vi "Couple Head Impulse Traces.vi"(0 "Data Input":T5 {"Data Channels" format="%.2f"}, 1 "Impulse Positions":T1(array[cluster]) {"Amplitude offset" format="%.2f"}, 2 "Trace Select":i32 min=0 max=1000, 3 "Impulse Direction +ve?":bool, 4 "Capture Saccade":bool, 5 "Impulse Plane":T4(ring), 6 "Mean and STD":bool, 7 "Plot Selection 2":T3 {"Gain" format="%.1f"; "Offset" format="%.1f"}, 8 "Export":bool, 9 "desacc":T2={"Threshold 1 [Acc]"=0.0, "Threshold 2 [% of TH1]"=0, "tolerance"=2, "Search WD "=0.05757575757575758, " always use TH2"=TRUE, "Range"=3.0303030303030303, "Max time"=50.0, "Min time"=1.0, "Velocity Threshold"=0} {"Velocity Threshold" scale=0.0..100.0; "Range" scale=0.0..5.0; "Search WD" scale=0.0..0.3; "tolerance" scale=0.0..10.0; "Threshold 2 [% of TH1]" scale=0.0..100.0; "Threshold 1 [Acc]" scale=1.0..20000.0}, 10 "Interpolate":bool, 13 "S-pline":bool, 15 "desacc.":bool=TRUE, 16 "man. desacc..":bool, 17 "Display Saccade":bool, 18 "balance parameter (s-pline Parameter)":dbl(slide)=0.9 min=0.8 max=1.0 step=0.0001 scale=0.8..1.0) -> (11 "Impulse Positions 2":T1(array[cluster]) {"Amplitude offset" format="%.2f"}, 12 "No Impulses":i32, 14 "Impulses":dbl[][](graph), 19 "Mean and STD":dbl[][](array[numeric]) format="%.2f")   [LabVIEW 2016, in "impulse functions.lvlib"]
uses:
  impulse functions.lvlib
  core/type-defs/TD_Impulse Parameter.ctl
  core/type-defs/TD_Impulse Planes.ctl
  <vilib>/Analysis/1siggen.llb/Ramp Pattern by Samples.vi
  stats/stats.lvlib
  <vilib>/Analysis/NI_AALPro.lvlib
  <vilib>/Analysis/NI_AALBase.lvlib
  core/core.lvlib
panel:
  out "Desaccaded 2":dbl[][](graph)
  # "Copyright Americo A. Migliaccio (c) 2002 All Rights Reserved by Author"
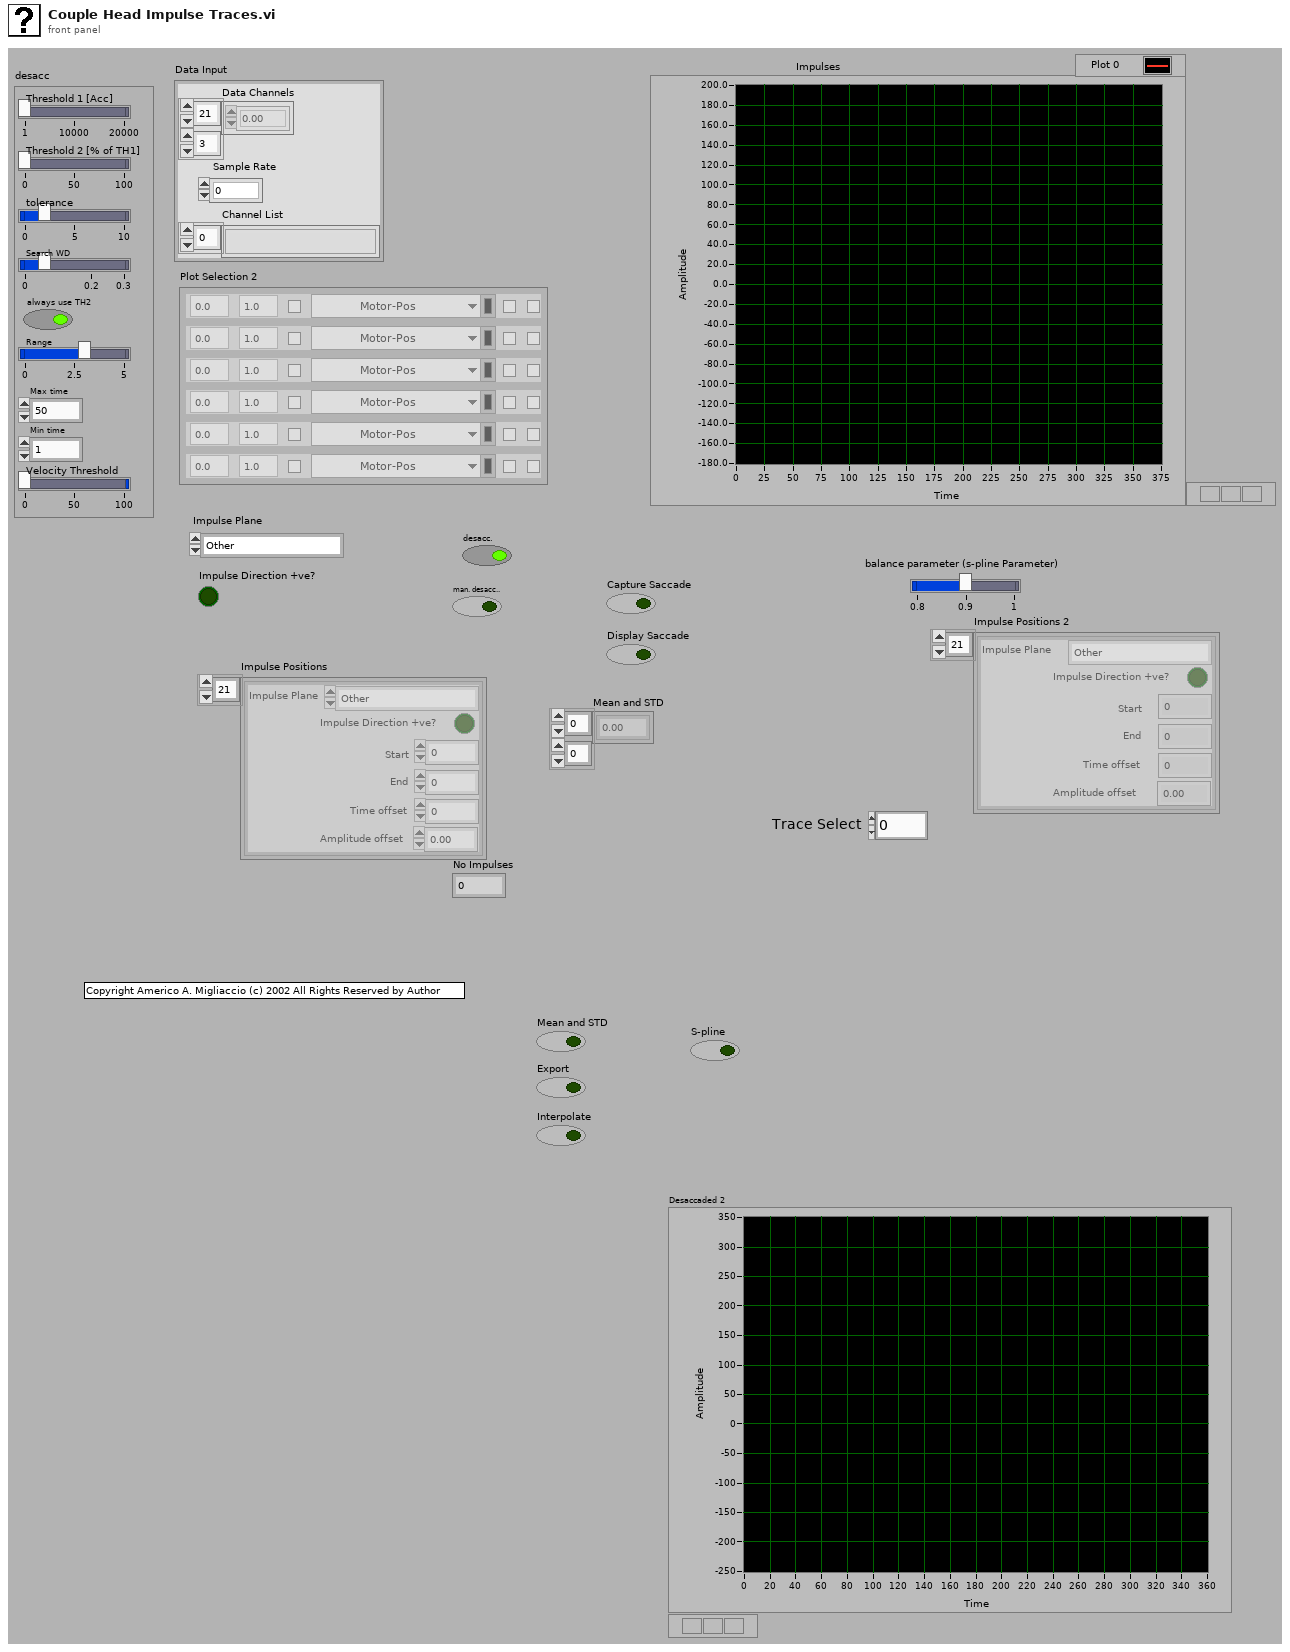
[diagram p1: front panel]
types:
  T1 = cluster{"Start":i32, "End":i32, "Impulse Plane":enum16{"Other", "Yaw", "Pitch", "Roll", "LARP", "RALP"}, "Impulse Direction +ve?":bool, "Time offset":i32, "Amplitude offset":dbl}[]
  T2 = cluster{"Threshold 1 [Acc]":dbl, "Threshold 2 [% of TH1]":i32, "tolerance":i32, "Search WD ":dbl, " always use TH2":bool, "Range":dbl, "Max time":dbl, "Min time":dbl, "Velocity Threshold":i32}
  T3 = typedef "core.lvlib/TD_Impulse Parameter.ctl" = cluster{"Color":u32, "Visible":bool, "Channel":u16, "Invert":bool, "Desaccade":bool, "Offset":dbl, "Gain":dbl}[]
  T4 = enum16{"Other", "Yaw", "Pitch", "Roll", "LARP", "RALP"}
  T5 = cluster{"Data Channels":dbl[][], "Sample Rate":i32, "Channel List":string[]}
  T6 = typedef "TD_Impulse Planes.ctl" = enum16{"Other", "Yaw", "Pitch", "Roll", "LARP", "RALP"}
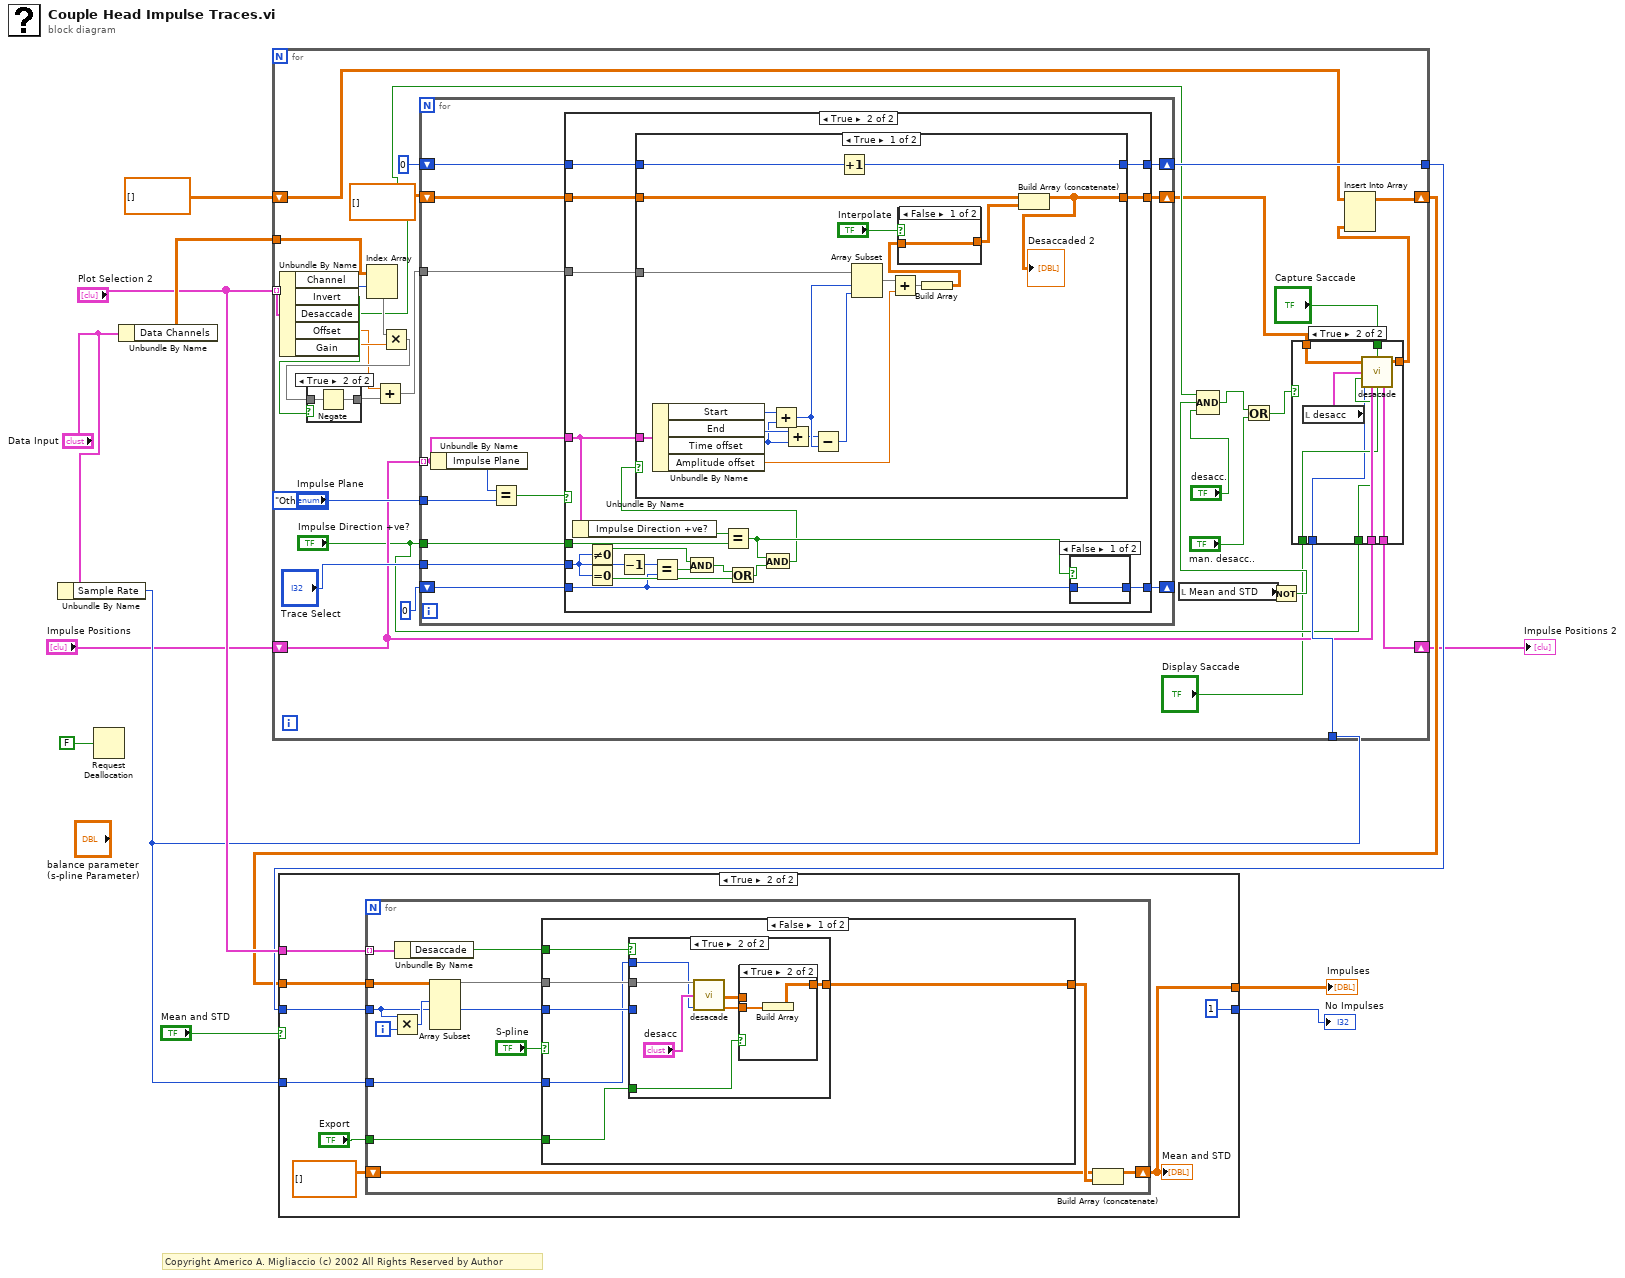
[diagram p0: block diagram]
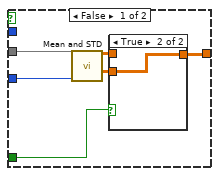
[diagram p3: hidden frame]
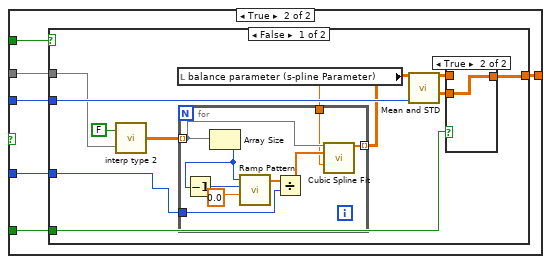
[diagram p6: hidden frame]
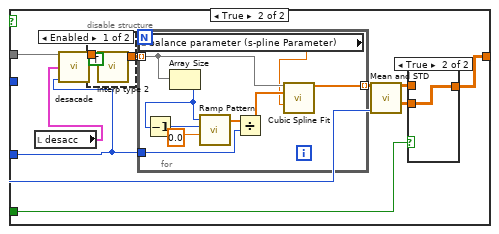
[diagram p8: hidden frame]
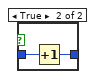
[diagram p14: hidden frame]
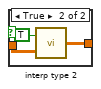
[diagram p15: hidden frame]
diagram:
  # "Copyright Americo A. Migliaccio (c) 2002 All Rights Reserved by Author"
  n1 = Unbundle By Name("Data Input") -> ("Sample Rate"=w6:i32)
  n2 = Request Deallocation(FALSE ("flag")) -> ()
  n3 = Unbundle By Name("Data Input") -> ("Data Channels"=w12:dbl[][])
  n4 = for {
    tunnel: "Plot Selection 2" -> [w43] mode=indexing
    shift-right: [w26] -> w7
    shift-left: dbl[][] [] -> [w28]
    tunnel: [w44] -> w10
    tunnel: w12 -> [w41]
    tunnel: w6 -> [w19]
    shift-right: [w17] -> w5
    shift-left: "Impulse Positions" -> [w18]
    (unwired) TD_Impulse_Planes."Other" ("Impulse Plane")
    n5 = Unbundle By Name(w43) -> ("Channel"=w42:u16, "Invert"=w38:bool, "Desaccade"=w30:bool, "Offset"=w34:dbl, "Gain"=w35:dbl)
    n6 = Index Array(array=w41, index (row)=w42) -> (element=w40:dbl[])  [unwired: 1 in]
    n7 = Multiply(x=w40, y=w35) -> (x*y=w39:dbl[])
    n8 = case shown="True" w38 {
      tunnel: w39 -> [w58 w60]
      tunnel: [w58 w59] -> w37
      frame False {
      }
      frame True {
        n9 = Negate(x=w60) -> (-x=w59:dbl[])
      }
    }
    n10 = Add(x=w34, y=w37) -> (x+y=w36:dbl[])
    n11 = for {
      tunnel: w18 -> [w71] mode=indexing
      tunnel: "Impulse Plane" -> [w72]
      tunnel: w36 -> [w70]
      shift-right: [w68] -> w29
      shift-left: dbl[][] [] -> [w69]
      tunnel: "Impulse Direction +ve?" -> [w67]
      shift-right: [w66] -> w44
      shift-left: 0 -> [w65]
      tunnel: "Trace Select" -> [w63]
      shift-right: [w61] -> _
      shift-left: 0 -> [w62]
      n12 = Unbundle By Name(w71) -> ("Impulse Plane"=w73:T4)
      n13 = Equal?(x=w73, y=w72) -> (x = y?=w64:bool)
      n14 = case shown="True" w64 {
        tunnel: w71 -> [_ w94]
        tunnel: w70 -> [_ w95]
        tunnel: w69 -> [w76 w93]
        tunnel: [w76 w92] -> w68
        tunnel: w67 -> [_ w91]
        tunnel: w65 -> [w75 w89]
        tunnel: [w75 w88] -> w66
        tunnel: w63 -> [_ w86]
        tunnel: w62 -> [w74 w82]
        tunnel: [w74 w87] -> w61
        frame False {
        }
        frame True {
          n15 = Unbundle By Name(w94) -> ("Impulse Direction +ve?"=w90:bool)
          n16 = Not Equal To 0?(x=w86) -> (x != 0?=w79:bool)
          n17 = Equal To 0?(x=w86) -> (x = 0?=w83:bool)
          n18 = Decrement(x=w86) -> (x-1=w81:i32)
          n19 = Equal?(x=w81, y=w82) -> (x = y?=w80:bool)
          n20 = And(x=w79, y=w80) -> (x .and. y?=w78:bool)
          n21 = Equal?(x=w90, y=w91) -> (x = y?=w85:bool)
          n22 = Or(x=w78, y=w83) -> (x .or. y?=w84:bool)
          n23 = And(x=w85, y=w84) -> (x .and. y?=w77:bool)
          n24 = case shown="True" w77 {
            tunnel: w94 -> [w116 _]
            tunnel: w95 -> [w113 _]
            tunnel: w93 -> [w112 w122]
            tunnel: [w99 w122] -> w92
            tunnel: w89 -> [w105 w121]
            tunnel: [w104 w121] -> w88
            frame True {
              n25 = Unbundle By Name(w116) -> ("Start"=w110:i32, "End"=w115:i32, "Time offset"=w108:i32, "Amplitude offset"=w106:dbl)
              n26 = Add(x=w110, y=w108) -> (x+y=w111:i32)
              n27 = Add(x=w115, y=w108) -> (x+y=w109:i32)
              n28 = Subtract(x=w109, y=w111) -> (x-y=w114:i32)
              n29 = Increment(x=w105) -> (x+1=w104:i32)
              n30 = Array Subset(array=w113, index=w111, length=w114) -> (w107:dbl[])
              n31 = Add(x=w107, y=w106) -> (x+y=w103:dbl[])
              n32 = Build Array(w103) -> (w102:dbl[][])
              n33 = case shown="False" "Interpolate" {
                tunnel: w102 -> [w117 w120]
                tunnel: [w117 w119] -> w100
                frame False {
                }
                frame True {
                  n34 = call "interp type 2.vi"("NaN"=w120, "Remove front and end"=TRUE) -> ("Interpolated"=w119:dbl[][])
                }
              }
              n35 = Build Array (concatenate)(w112, w100) -> (w99:dbl[][])
              "Desaccaded 2" <- w99
            }
            frame False {
            }
          }
          n36 = case shown="False" w85 {
            tunnel: w82 -> [w96 w98]
            tunnel: [w96 w97] -> w87
            frame False {
            }
            frame True {
              n37 = Increment(x=w98) -> (x+1=w97:i32)
            }
          }
        }
      }
    }
    n38 = local read "Mean and STD"() -> (w31:bool)
    n39 = Not(x=w31) -> (.not. x?=w24:bool)
    n40 = Compound Arithmetic op=AND(w30, w24, "desacc.") -> (w21:bool)
    n41 = Or(x=w21, y="man. desacc..") -> (x .or. y?=w20:bool)
    n42 = case shown="True" w20 {
      tunnel: [w48 w57] -> w27
      tunnel: w29 -> [w48 w50]
      tunnel: w19 -> [_ w49]
      tunnel: w18 -> [w47 w55]
      tunnel: [w47 w54] -> w17
      tunnel: "Display Saccade" -> [_ w53]
      tunnel: "Impulse Direction +ve?" -> [_ w52]
      tunnel: "Capture Saccade" -> [_ w51]
      frame False {
      }
      frame True {
        n43 = local read "desacc"() -> (w56:T2)
        n44 = call "desacade.vi"("Data not diff"=w50, "Capture Saccades"=w51, "desacc"=w56, "Impulse Direction +ve?"=w52, "Sample Rate"=w49, "Impulse Positions"=w55, "Display Saccades"=w53) -> ("Desaccaded"=w57:dbl[][], "Impulse Positions 2"=w54:T1)  [unwired: 3 in, 4 out]
      }
    }
    n45 = Insert Into Array(array=w28, new element=w27) -> (w26:dbl[][])  [unwired: 2 in]
  }
  "Impulse Positions 2" <- w5
  n46 = case shown="True" "Mean and STD" {
    tunnel: "Plot Selection 2" -> [_ w132]
    tunnel: w7 -> [w124 w131]
    tunnel: w10 -> [w123 w130]
    tunnel: w6 -> [_ w127]
    tunnel: [w124 w126] -> w4
    tunnel: [w123 1] -> w3
    frame False {
    }
    frame True {
      n47 = for {
        tunnel: w132 -> [w145] mode=indexing
        tunnel: w131 -> [w143]
        tunnel: w130 -> [w139]
        shift-right: [w137] -> w126
        shift-left: dbl[][] [] -> [w136]
        tunnel: "Export" -> [w135]
        tunnel: w127 -> [w133]
        i -> [w142]
        n48 = Multiply(x=w139, y=w142) -> (x*y=w141:i32)
        n49 = Unbundle By Name(w145) -> ("Desaccade"=w144:bool)
        n50 = Array Subset(array=w143, index (row)=w141, length (row)=w139) -> (w140:dbl[][])  [unwired: 2 in]
        n51 = case shown="False" "S-pline" {
          tunnel: w144 -> [w151 w175]
          tunnel: w140 -> [w150 w174]
          tunnel: w139 -> [w149 w173]
          tunnel: [w148 w172] -> w138
          tunnel: w135 -> [w147 w171]
          tunnel: w133 -> [w146 w170]
          frame False {
            n52 = case shown="True" w151 {
              tunnel: w150 -> [w152 w166]
              tunnel: w149 -> [w157 _]
              tunnel: [w153 w163] -> w148
              tunnel: w147 -> [w154 w162]
              tunnel: w146 -> [_ w160]
              frame False {
                n53 = call "Mean and STD.vi"("Data (in)"=w152, "Number of Impulses"=w157) -> ("Mean and STD"=w155:dbl[][], "Mean"=w156:dbl[][])  [unwired: 11 in, 1 out]
                n54 = case shown="True" w154 {
                  tunnel: w156 -> [_ w159]
                  tunnel: [w158 w159] -> w153
                  tunnel: w155 -> [w158 _]
                  frame False {
                  }
                  frame True {
                  }
                }
              }
              frame True {
                n55 = call "desacade.vi"("Data not diff"=w166, "desacc"="desacc", "Sample Rate"=w160) -> ("Mean and STD"=w164:dbl[][], "Mean (-inf)"=w165:dbl[])  [unwired: 7 in, 4 out]
                n56 = case shown="True" w162 {
                  tunnel: w165 -> [_ w169]
                  tunnel: w164 -> [w167 _]
                  tunnel: [w167 w168] -> w163
                  frame False {
                  }
                  frame True {
                    n57 = Build Array(w169) -> (w168:dbl[][])
                  }
                }
              }
            }
          }
          frame True {
            n58 = case shown="False" w175 {
              tunnel: w174 -> [w180 w208]
              tunnel: w173 -> [w186 w203]
              tunnel: [w182 w201] -> w172
              tunnel: w171 -> [w183 w200]
              tunnel: w170 -> [w177 w198]
              frame False {
                n59 = call "interp type 2.vi"("NaN"=w180, "Remove front and end"=FALSE) -> ("Interpolated"=w181:dbl[][])
                n60 = local read "balance parameter (s-pline Parameter)"() -> (w178:dbl)
                n61 = for {
                  tunnel: w177 -> [w189]
                  tunnel: w181 -> [w192] mode=indexing
                  tunnel: [w191] -> w179 mode=indexing
                  tunnel: w178 -> [w187]
                  n62 = Array Size(array=w192) -> (size(s)=w194:i32)
                  n63 = Decrement(x=w194) -> (x-1=w193:i32)
                  n64 = call-poly <vilib>:"Ramp Pattern.vi"("start"=0.0, "end"=w193, "samples"=w194) -> ("Ramp Pattern"=w190:dbl[])  [unwired: 7 in, 1 out]
                  n65 = Divide(x=w190, y=w189) -> (x/y=w188:dbl[])
                  n66 = call <vilib>:"Cubic Spline Fit.vi"("Y"=w192, "X"=w188, "balance parameter"=w187) -> ("Best Cubic Spline Fit"=w191:dbl[])  [unwired: 11 in, 1 out]
                }
                n67 = call "Mean and STD.vi"("Data (in)"=w179, "Number of Impulses"=w186) -> ("Mean and STD"=w184:dbl[][], "Mean"=w185:dbl[][])  [unwired: 11 in, 1 out]
                n68 = case shown="True" w183 {
                  tunnel: w185 -> [_ w197]
                  tunnel: [w196 w197] -> w182
                  tunnel: w184 -> [w196 _]
                  frame False {
                  }
                  frame True {
                  }
                }
              }
              frame True {
                n69 = local read "desacc"() -> (w199:T2)
                n70 = call "desacade.vi"("Data not diff"=w208, "desacc"=w199, "Sample Rate"=w198) -> ("Desaccaded"=w207:dbl[][])  [unwired: 7 in, 5 out]
                n71 = disable-structure shown="Enabled" {
                  disable-tunnel: w207 -> [w211 w212]
                  disable-tunnel: [w210 w212] -> w206
                  frame Enabled {
                    n72 = call "interp type 2.vi"("NaN"=w211, "Remove front and end"=TRUE) -> ("Interpolated"=w210:dbl[][])
                  }
                  frame Disabled {
                  }
                }
                n73 = for {
                  tunnel: w198 -> [w217]
                  tunnel: w206 -> [w220] mode=indexing
                  tunnel: [w219] -> w202 mode=indexing
                  n74 = local read "balance parameter (s-pline Parameter)"() -> (w215:dbl)
                  n75 = Array Size(array=w220) -> (size(s)=w222:i32)
                  n76 = Decrement(x=w222) -> (x-1=w221:i32)
                  n77 = call-poly <vilib>:"Ramp Pattern.vi"("start"=0.0, "end"=w221, "samples"=w222) -> ("Ramp Pattern"=w218:dbl[])  [unwired: 7 in, 1 out]
                  n78 = Divide(x=w218, y=w217) -> (x/y=w216:dbl[])
                  n79 = call <vilib>:"Cubic Spline Fit.vi"("Y"=w220, "X"=w216, "balance parameter"=w215) -> ("Best Cubic Spline Fit"=w219:dbl[])  [unwired: 11 in, 1 out]
                }
                n80 = call "Mean and STD.vi"("Data (in)"=w202, "Number of Impulses"=w203) -> ("Mean and STD"=w205:dbl[][], "Mean"=w204:dbl[][])  [unwired: 11 in, 1 out]
                n81 = case shown="True" w200 {
                  tunnel: w204 -> [_ w214]
                  tunnel: [w213 w214] -> w201
                  tunnel: w205 -> [w213 _]
                  frame False {
                  }
                  frame True {
                  }
                }
              }
            }
          }
        }
        n82 = Build Array (concatenate)(w136, w138) -> (w137:dbl[][])
      }
      "Mean and STD" <- w126
    }
  }
  "Impulses" <- w4
  "No Impulses" <- w3
